vi "SFC_Get Output ATest Data.vi"(0 "Traceability 引用句柄":refnum<k24>, 1 "ExtSerialNo":string, 2 "DateTo":string, 5 "Model":string, 7 "PalletID":string, 9 "CartonID":string, 11 "error in (no error)":errorcluster caption="错误输入（无错误）", 12 "DateFrom":string, 13 "tblName":string) -> (4 "Traceability 引用句柄输出":refnum<k24>, 6 ".NET:System.Data.DataSet":T1={"CaseSensitive"=FALSE, "Container"=refnum, "DataSetName"="", "DefaultViewManager"=refnum, "DesignMode"=FALSE, "EnforceConstraints"=FALSE, "ExtendedProperties"=refnum, "HasErrors"=FALSE, "IsInitialized"=FALSE, "Locale"=refnum, "Namespace"="", "Prefix"="", "Relations"=refnum, "RemotingFormat"=0, "SchemaSerializationMode"=1, "Site"=refnum, "Tables"=refnum} {"SchemaSerializationMode" items=["IncludeSchema"=1, "ExcludeSchema"=2]; "RemotingFormat" items=["Xml", "Binary"]}, 15 "error out":errorcluster caption="错误输出")   [LabVIEW 2014, in "Traceability.lvlib"]
uses:
  D:/webservice/Traceability.dll
  Traceability.dll
  System.Data
  Traceability.lvlib
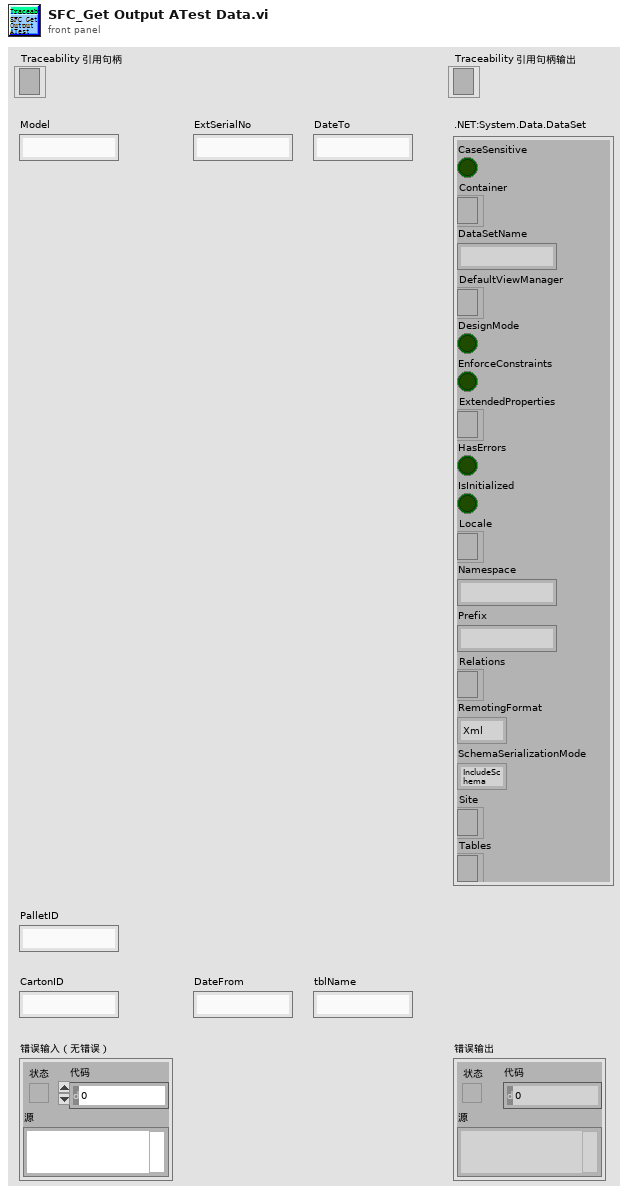
[diagram p1: front panel]
types:
  T1 = cluster{"CaseSensitive":bool, "Container":refnum<k24>, "DataSetName":string, "DefaultViewManager":refnum<k24>, "DesignMode":bool, "EnforceConstraints":bool, "ExtendedProperties":refnum<k24>, "HasErrors":bool, "IsInitialized":bool, "Locale":refnum<k24>, "Namespace":string, "Prefix":string, "Relations":refnum<k24>, "RemotingFormat":i32, "SchemaSerializationMode":i32, "Site":refnum<k24>, "Tables":refnum<k24>}
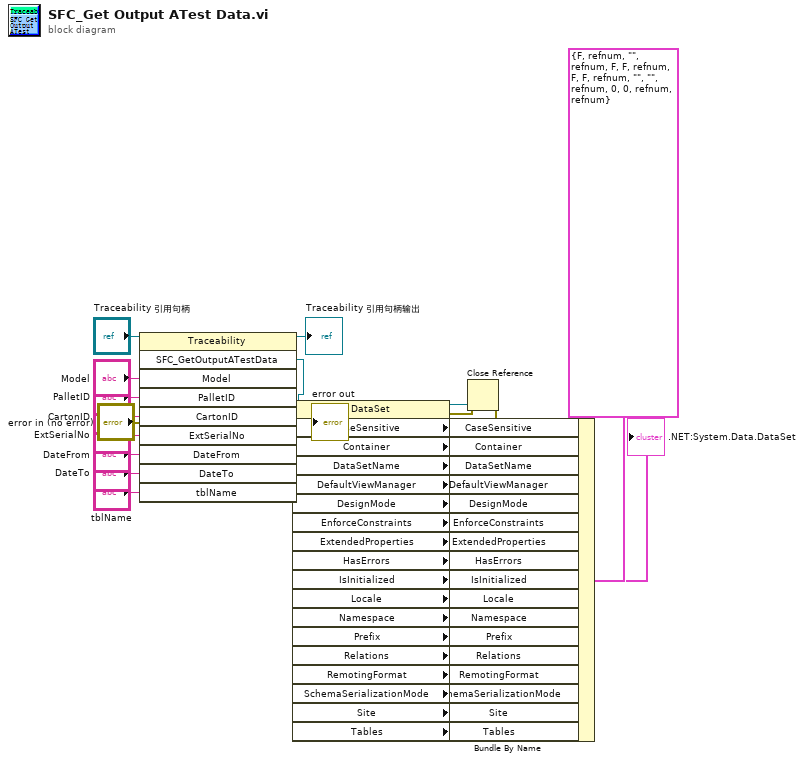
[diagram p0: block diagram]
diagram:
  n1 = invoke class="Traceability" method="SFC_GetOutputATestData"(reference="Traceability 引用句柄", error in="error in (no error)", "Model"="Model", "PalletID"="PalletID", "CartonID"="CartonID", "ExtSerialNo"="ExtSerialNo", "DateFrom"="DateFrom", "DateTo"="DateTo", "tblName"="tblName") -> (reference out=→"Traceability 引用句柄输出":refnum<k24>, error out=w4:errorcluster, "SFC_GetOutputATestData"=w31:refnum<k24>)  [unwired: 1 in, 7 out]
  n2 = property class="DataSet"(reference=w31, error in=w4) -> (reference out=w3:refnum<k24>, error out=w2:errorcluster, "CaseSensitive"=w28:bool, "Container"=w27:refnum<k24>, "DataSetName"=w26:string, "DefaultViewManager"=w25:refnum<k24>, "DesignMode"=w24:bool, "EnforceConstraints"=w23:bool, "ExtendedProperties"=w22:refnum<k24>, "HasErrors"=w21:bool, "IsInitialized"=w20:bool, "Locale"=w19:refnum<k24>, "Namespace"=w18:string, "Prefix"=w17:string, "Relations"=w16:refnum<k24>, "RemotingFormat"=w15:i32, "SchemaSerializationMode"=w14:i32, "Site"=w13:refnum<k24>, "Tables"=w12:refnum<k24>)
  n3 = Bundle By Name(cluster=T1 {"CaseSensitive"=FALSE, "Container"=refnum, "DataSetName"="", "DefaultViewManager"=refnum, "DesignMode"=FALSE, "EnforceConstraints"=FALSE, "ExtendedProperties"=refnum, "HasErrors"=FALSE, "IsInitialized"=FALSE, "Locale"=refnum, "Namespace"="", "Prefix"="", "Relations"=refnum, "RemotingFormat"=0, "SchemaSerializationMode"=0, "Site"=refnum, "Tables"=refnum} (".NET:System.Data.DataSet"), "CaseSensitive"=w28, "Container"=w27, "DataSetName"=w26, "DefaultViewManager"=w25, "DesignMode"=w24, "EnforceConstraints"=w23, "ExtendedProperties"=w22, "HasErrors"=w21, "IsInitialized"=w20, "Locale"=w19, "Namespace"=w18, "Prefix"=w17, "Relations"=w16, "RemotingFormat"=w15, "SchemaSerializationMode"=w14, "Site"=w13, "Tables"=w12) -> (→".NET:System.Data.DataSet":T1)
  n4 = Close Reference(reference=w3, error in (no error)=w2) -> (error out=→"error out":errorcluster)
